vi "Control Info.vi"(8 "error in (no error)":errorcluster, 10 "Control Type":string, 11 "Control List in":refnum<class "Control List.lvclass">) -> (0 "error out":errorcluster, 2 "Control Info":T1, 3 "Control List out":refnum<class "Control List.lvclass">)   [LabVIEW 2020, in "VolatusGUIEditor.lvlib" / "Control List.lvclass"]
uses:
  Control List.lvclass
  Control List.lvclass/Control List.ctl
  <vilib>/picture/picture.llb/imagedata.ctl
  Control Info.ctl
  VolatusGUIEditor.lvlib
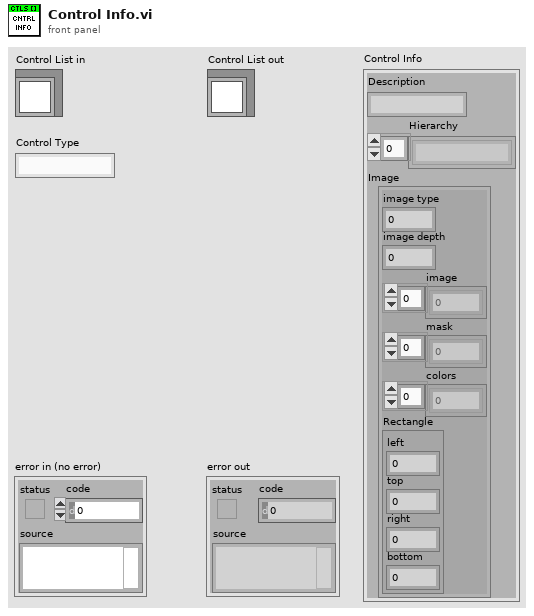
[diagram p1: front panel]
types:
  T1 = typedef "VolatusGUIEditor.lvlib/Control Info.ctl" = cluster{"Description":string, "Hierarchy":string[], "Image":T2}
  T2 = typedef "imagedata.ctl" = cluster{"image type":i32, "image depth":i32, "image":u8[], "mask":u8[], "colors":u32[], "Rectangle":cluster{"left":i16, "top":i16, "right":i16, "bottom":i16}}
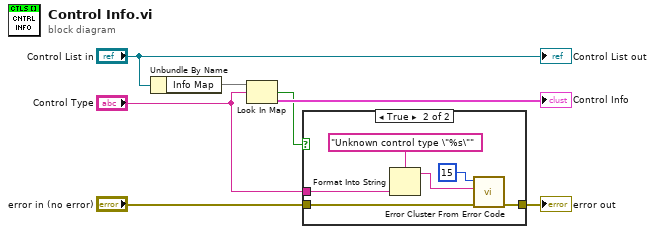
[diagram p0: block diagram]
diagram:
  n1 = Unbundle By Name("Control List in") -> ("Info Map"=w6:map{string, T1})
  n2 = Look In Map(map=w6, key="Control Type") -> (key not found?=w3:bool, value=→"Control Info":T1)  [unwired: 1 in]
  n3 = case shown="True" w3 {
    tunnel: "error in (no error)" -> [w8 w12]
    tunnel: "Control Type" -> [_ w14]
    tunnel: [w8 w9] -> w1
    frame False {
    }
    frame True {
      n4 = Format Into String(format string="Unknown control type \"%s\"", w14) -> (resulting string=w11:string)  [unwired: 2 in, 1 out]
      n5 = call <vilib>:"Error Cluster From Error Code.vi"("error in (no error)"=w12, "error message (\"\")"=w11, "error code (0)"=15) -> ("error out"=w9:errorcluster)  [unwired: 6 in]
    }
  }
  "error out" <- w1
  "Control List out" <- "Control List in"
